vi "right shift.vi"(11 "2048 2":dbl[][](array[numeric])) -> (3 "2048":dbl[][](array[numeric]))   [LabVIEW 2015]
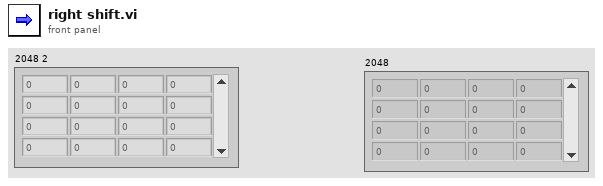
[diagram p1: front panel]
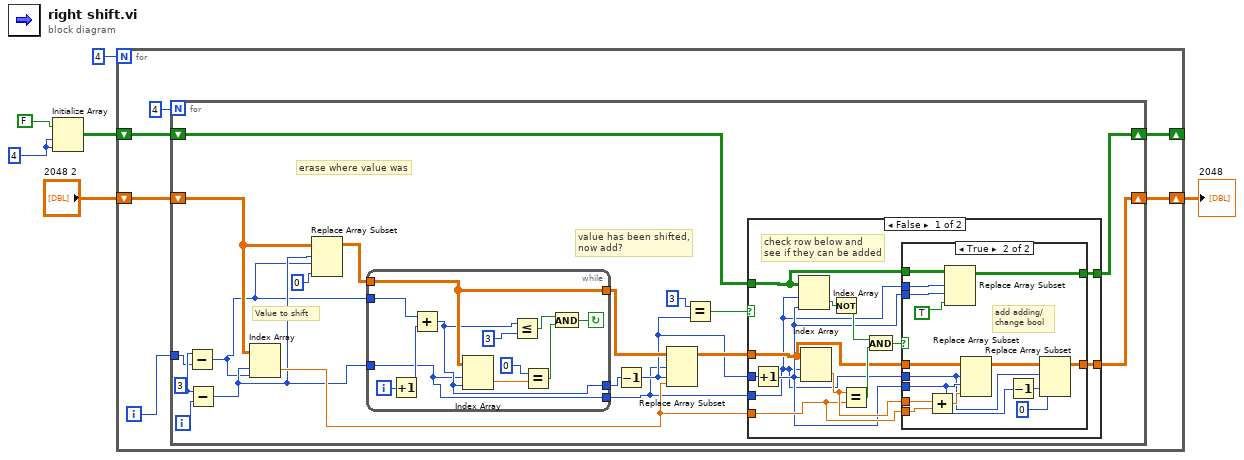
[diagram p0: block diagram]
diagram:
  w3 = 4
  n1 = Initialize Array(FALSE, w3, w3) -> (w1:bool[][])
  n2 = for {
    N: 4 -> [_]
    shift-right: [w8] -> _
    shift-left: w1 -> [w9]
    shift-right: [w7] -> w4
    shift-left: "2048 2" -> [w11]
    i -> [w10]
    n3 = for {
      N: 4 -> [_]
      tunnel: w10 -> [w15]
      shift-right: [w24] -> w8
      shift-left: w9 -> [w25]
      shift-right: [w23] -> w7
      shift-left: w11 -> [w21]
      i -> [w19]
      w16 = 3
      # "erase where value was"
      # "value has been shifted,\nnow add?"
      # "Value to shift"
      n4 = Subtract(x=w16, y=w15) -> (x-y=w17:i32)
      n5 = Subtract(x=w16, y=w19) -> (x-y=w18:i32)
      n6 = Index Array(array=w21, index (row)=w18, index (col)=w17) -> (element=w26:dbl)
      n7 = Replace Array Subset(array=w21, new element=0, index (row)=w18, index (col)=w17) -> (w22:dbl[][])
      n8 = while {
        tunnel: w17 -> [w75]
        tunnel: w18 -> [w65]
        tunnel: w22 -> [w67]
        tunnel: [w65] -> w13
        tunnel: [w66] -> w27
        tunnel: [w67] -> w31
        i -> [w74]
        stop <- w70 continue-if-true
        n9 = Increment(x=w74) -> (x+1=w71:i32)
        n10 = Add(x=w75, y=w71) -> (x+y=w66:i32)
        n11 = Index Array(array=w67, index (row)=w65, index (col)=w66) -> (element=w73:dbl)
        n12 = Less Or Equal?(x=w66, y=3) -> (x <= y?=w68:bool)
        n13 = Equal?(x=0, y=w73) -> (x = y?=w72:bool)
        n14 = And(x=w68, y=w72) -> (x .and. y?=w70:bool)
      }
      n15 = Decrement(x=w27) -> (x-1=w14:i32)
      n16 = Replace Array Subset(array=w31, new element=w26, index (row)=w13, index (col)=w14) -> (w28:dbl[][])
      n17 = Equal?(x=3, y=w14) -> (x = y?=w29:bool)
      n18 = case shown="False" w29 {
        tunnel: w28 -> [w38 w62]
        tunnel: w13 -> [w32 _]
        tunnel: w14 -> [w44 _]
        tunnel: w26 -> [w36 _]
        tunnel: w25 -> [w40 w63]
        tunnel: [w35 w63] -> w24
        tunnel: [w34 w62] -> w23
        frame False {
          # "check row below and \nsee if they can be added"
          n19 = Increment(x=w44) -> (x+1=w33:i32)
          n20 = Index Array(array=w40, index (row)=w32, index (col)=w33) -> (element=w42:bool)
          n21 = Index Array(array=w38, index (row)=w32, index (col)=w33) -> (element=w37:dbl)
          n22 = Not(x=w42) -> (.not. x?=w41:bool)
          n23 = Equal?(x=w37, y=w36) -> (x = y?=w43:bool)
          n24 = And(x=w41, y=w43) -> (x .and. y?=w39:bool)
          n25 = case shown="True" w39 {
            tunnel: w40 -> [w46 w61]
            tunnel: w33 -> [_ w60]
            tunnel: w32 -> [_ w59]
            tunnel: w38 -> [w45 w57]
            tunnel: w32 -> [_ w47]
            tunnel: w33 -> [_ w49]
            tunnel: w37 -> [_ w55]
            tunnel: w36 -> [_ w54]
            tunnel: [w46 w53] -> w35
            tunnel: [w45 w51] -> w34
            frame False {
            }
            frame True {
              # "add adding/\nchange bool"
              n26 = Add(x=w55, y=w54) -> (x+y=w56:dbl)
              n27 = Replace Array Subset(array=w61, new element=TRUE, index (row)=w59, index (col)=w60) -> (w53:bool[][])
              n28 = Replace Array Subset(array=w57, new element=w56, index (row)=w47, index (col)=w49) -> (w52:dbl[][])
              n29 = Decrement(x=w49) -> (x-1=w48:i32)
              n30 = Replace Array Subset(array=w52, new element=0, index (row)=w47, index (col)=w48) -> (w51:dbl[][])
            }
          }
        }
        frame True {
          # "if it is row 0 then,\n no adds to check"
        }
      }
    }
  }
  "2048" <- w4
